vi "WaitOnBoardSettings.vi"(8 "error in (no error)":errorcluster, 11 "KST101 in":refnum<class "KST101.lvclass">) -> (0 "error out":errorcluster, 3 "KST101 out":refnum<class "KST101.lvclass">)   [LabVIEW 2016, in "Stepper Motor Controller.lvlib" / "KST101.lvclass"]
uses:
  KST101.lvclass
  KST101.lvclass/KST101.ctl
  D:/Workspace/ProCyteOne_LaserModuleAlignment/shared/Thorlabs/Kinesis/Dependencies/Thorlabs.MotionControl.KCube.StepperMotorCLI.dll
  Dependencies/Thorlabs.MotionControl.KCube.StepperMotorCLI.dll
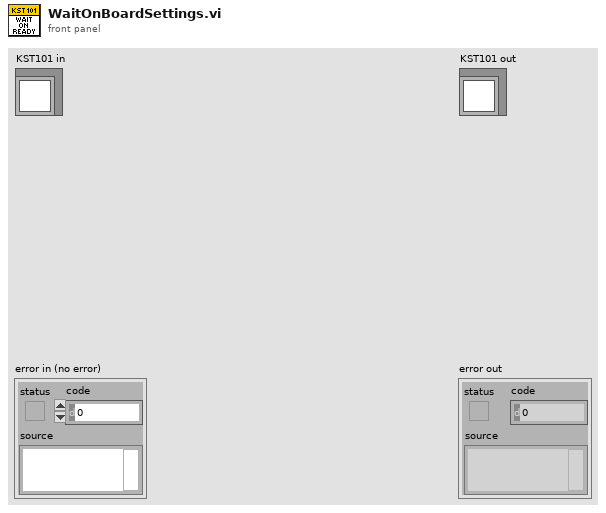
[diagram p1: front panel]
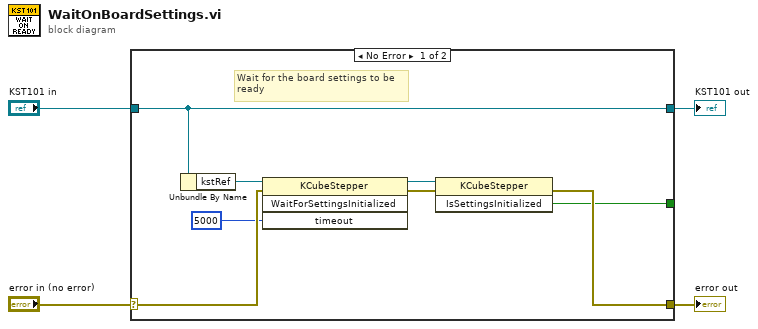
[diagram p0: block diagram]
diagram:
  n1 = case shown="No Error" "error in (no error)" {
    selector: "error in (no error)" -> [w11 w14]
    tunnel: [w6 w14] -> w3
    tunnel: [w12 w13] -> w1
    tunnel: "KST101 in" -> [w12 w13]
    tunnel: [w5 _] -> _
    frame No Error {
      # "Wait for the board settings to be\nready"
      n2 = Unbundle By Name(w12) -> ("kstRef"=w10:refnum<k24>)
      n3 = invoke class="KCubeStepper" method="WaitForSettingsInitialized"(reference=w10, error in=w11, "timeout"=5000) -> (reference out=w8:refnum<k24>, error out=w7:errorcluster)  [unwired: 1 in, 2 out]
      n4 = invoke class="KCubeStepper" method="IsSettingsInitialized"(reference=w8, error in=w7) -> (error out=w6:errorcluster, "IsSettingsInitialized"=w5:bool)  [unwired: 1 in, 1 out]
    }
    frame Error {
    }
  }
  "error out" <- w3
  "KST101 out" <- w1
